vi "Orca Data Spooler Modify Destination.vi"(0 "Destination":path, 11 "Source":path, 13 "Ignore Source?":bool) -> (4 "Modified Destination":path)   [LabVIEW 2020]
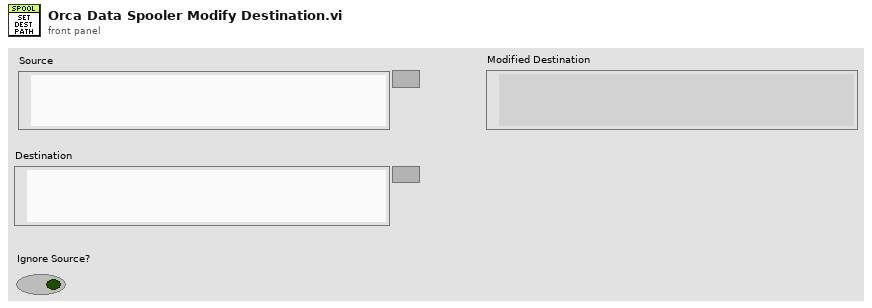
[diagram p1: front panel]
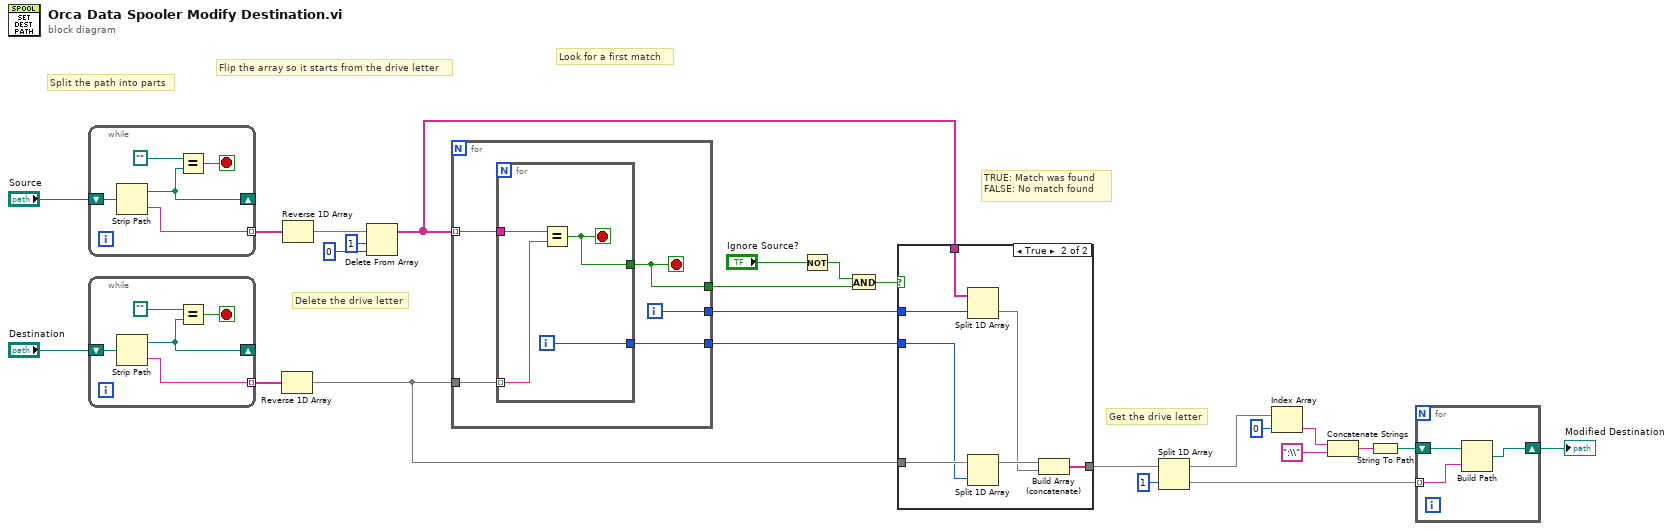
[diagram p0: block diagram]
diagram:
  # "Get the drive letter"
  # "TRUE: Match was found\nFALSE: No match found"
  # "Look for a first match"
  # "Delete the drive letter"
  # "Split the path into parts"
  # "Flip the array so it starts from the drive letter"
  n1 = while {
    tunnel: [w26] -> w23 mode=indexing
    shift-right: [w27] -> _
    shift-left: "Source" -> [w28]
    stop <- w29 stop-if-true
    n2 = Strip Path(path=w28) -> (stripped path=w27:path, name=w26:string)
    n3 = Equal?(x=path "", y=w27) -> (x = y?=w29:bool)
  }
  n4 = while {
    tunnel: [w31] -> w22 mode=indexing
    shift-right: [w32] -> _
    shift-left: "Destination" -> [w33]
    stop <- w34 stop-if-true
    n5 = Strip Path(path=w33) -> (stripped path=w32:path, name=w31:string)
    n6 = Equal?(x=path "", y=w32) -> (x = y?=w34:bool)
  }
  n7 = Reverse 1D Array(array=w22) -> (reversed array=w18:string[])
  n8 = Reverse 1D Array(array=w23) -> (reversed array=w21:string[])
  n9 = Delete From Array(array=w21, length=1, index=0) -> (array with subset deleted=w16:string[])  [unwired: 1 out]
  n10 = for {
    tunnel: w16 -> [w40] mode=indexing
    tunnel: w18 -> [w39]
    tunnel: [w38] -> w17
    tunnel: [w37] -> w15
    tunnel: [w36] -> w13
    i -> [w37]
    stop <- w36 stop-if-true
    n11 = for {
      tunnel: w40 -> [w44]
      tunnel: w39 -> [w43] mode=indexing
      tunnel: [w42] -> w36
      tunnel: [w41] -> w38
      i -> [w41]
      stop <- w42 stop-if-true
      n12 = Equal?(x=w44, y=w43) -> (x = y?=w42:bool)
    }
  }
  n13 = Not(x="Ignore Source?") -> (.not. x?=w11:bool)
  n14 = And(x=w11, y=w13) -> (x .and. y?=w12:bool)
  n15 = case shown="True" w12 {
    tunnel: w18 -> [w45 w52]
    tunnel: w17 -> [_ w51]
    tunnel: w16 -> [_ w50]
    tunnel: w15 -> [_ w49]
    tunnel: [w45 w46] -> w10
    frame False {
    }
    frame True {
      n16 = Split 1D Array(array=w50, index=w49) -> (second subarray=w47:string[])  [unwired: 1 out]
      n17 = Split 1D Array(array=w52, index=w51) -> (first subarray=w48:string[])  [unwired: 1 out]
      n18 = Build Array (concatenate)(w48, w47) -> (w46:string[])
    }
  }
  n19 = Split 1D Array(array=w10, index=1) -> (first subarray=w8:string[], second subarray=w2:string[])
  n20 = Index Array(array=w8, index=0) -> (element=w6:string)
  n21 = Concatenate Strings(w6, ":\\") -> (w4:string)
  n22 = String To Path(string=w4) -> (path=w3:path)
  n23 = for {
    shift-right: [w54] -> w1
    shift-left: w3 -> [w55]
    tunnel: w2 -> [w53] mode=indexing
    n24 = Build Path(base path=w55, name or relative path=w53) -> (appended path=w54:path)
  }
  "Modified Destination" <- w1
